vi "Move.vi"(8 "error in (no error)":errorcluster, 11 "XRay Scene in":refnum<class "XRay Scene.lvclass">=refnum) -> (0 "error out":errorcluster, 2 "Scene Object":refnum<vi>, 3 "XRay Scene out":refnum<class "XRay Scene.lvclass">)   [LabVIEW 2026, in "XRay Scene.lvclass"]
uses:
  XRay Scene.lvclass
  XRay Cabinet/XRay Cabinet.lvclass
  XRay Axis Rails/XRay Axis Rails.lvclass
  XRay CArm/XRay CArm.lvclass
  XRay Table/XRay Table.lvclass
  XRay Scene.lvclass/XRay Scene.ctl
  f3a4ce1a-163d-418c-9a4d-74df9f9edd9a.vi
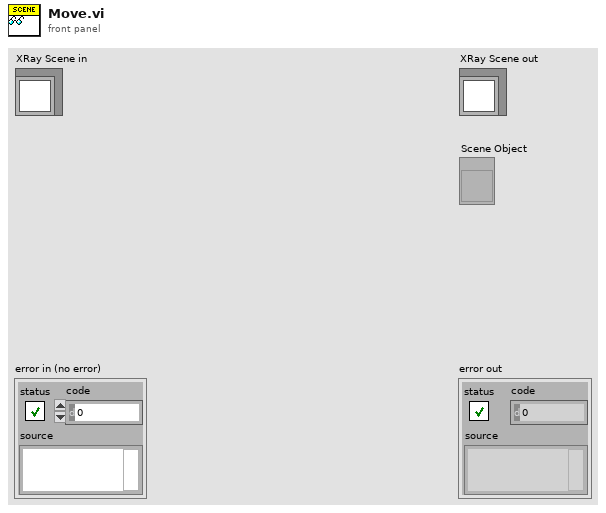
[diagram p1: front panel]
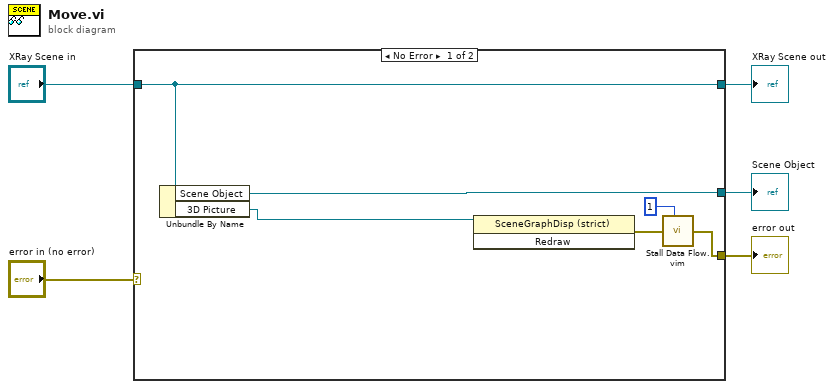
[diagram p0: block diagram]
diagram:
  n1 = case shown="No Error" "error in (no error)" {
    selector: "error in (no error)" -> [_ w12]
    tunnel: [w7 w12] -> w4
    tunnel: [w9 w13] -> w2
    tunnel: "XRay Scene in" -> [w9 w13]
    tunnel: [w11 _] -> w1
    frame No Error {
      n2 = Unbundle By Name(w9) -> ("Scene Object"=w11:refnum<vi>, "3D Picture"=w10:refnum<vi>)
      n3 = invoke class="SceneGraphDisp (strict)" method="Redraw"(reference=w10) -> (error out=w8:errorcluster)  [unwired: 2 in, 2 out]
      n4 = call "Stall Data Flow.vim"("value in"=w8, "milliseconds to wait"=u32 1) -> ("value out"=w7:errorcluster)  [unwired: 1 out]
    }
    frame Error {
    }
  }
  "error out" <- w4
  "XRay Scene out" <- w2
  "Scene Object" <- w1
